vi "WPI_IMU_ADIS16448_HardwareResetDelay.vi"(7 "Delay (ms)":u32=5000, 8 "error in":errorcluster, 11 "DigitalOutputDevRef":T1={"DIO Channel"=enum."DIO 1", "DevStatus"={"status"=FALSE, "code"=0, "source"=""}}) -> (0 "error out":errorcluster, 3 "DigitalOutputDevRef":T1={"DIO Channel"=enum."DIO 1", "DevStatus"={"status"=FALSE, "code"=0, "source"=""}})   [LabVIEW 2015, in "Apple Pi Gyro Library.lvlib" / "FRC_ADIS16448_IMU.lvlib"]
uses:
  FRC_ADIS16448_IMU.lvlib
  <vilib>/Rock Robotics/WPI/DigitalOutput/WPI_DigitalOutputDevRef.ctl
  <vilib>/Rock Robotics/SystemInterfaces/DIO/FPGA_DIOChannel.ctl
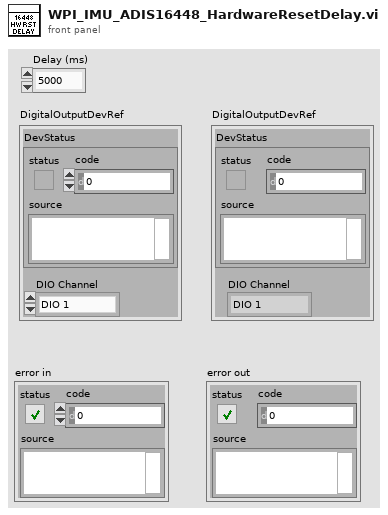
[diagram p1: front panel]
types:
  T1 = typedef "WPI_DigitalOutputDevRef.ctl" = cluster{"DIO Channel":T2, "DevStatus":errorcluster}
  T2 = typedef "FPGA_DIOChannel.ctl" = enum8{"DIO 0", "DIO 1", "DIO 2", "DIO 3", "DIO 4", "DIO 5", "DIO 6", "DIO 7", "DIO 8", "DIO 9", "DIO MXP 0", "DIO MXP 1", "DIO MXP 2", "DIO MXP 3", "DIO MXP 4", "DIO MXP 5", "DIO MXP 6", "DIO MXP 7", "DIO MXP 8", "DIO MXP 9", "DIO MXP 10", "DIO MXP 11", "DIO MXP 12", "DIO MXP 13", "DIO MXP 14", "DIO MXP 15", "Invalid"}
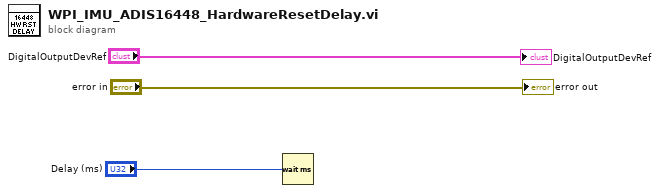
[diagram p0: block diagram]
diagram:
  n1 = Wait (ms)(milliseconds to wait="Delay (ms)") -> ()  [unwired: 1 out]
  "error out" <- "error in"
  "DigitalOutputDevRef" <- "DigitalOutputDevRef"
